vi "AlliGator Load Single Gate Image from .bin File.vi"(6 "Action":T1, 8 "error in (no error)":errorcluster, 10 "File Info":variant, 11 "Gate Index":i32) -> (0 "error out":errorcluster, 1 "Data 2":sgl[][](array[numeric]), 3 "Data 1":sgl[][](array[numeric]))   [LabVIEW 2021, in "AlliGator Files.lvlib"]
doc: "Single gate image loading step for PicoQuant .bin files."
uses:
  AlliGator Files.lvlib
  AlliGator FLI Image Stack Action.ctl
  PicoQuant/BIN/Extended PQ .bin Dataset Information.ctl
  PicoQuant/BIN/BIN File Information.ctl
  PicoQuant/PicoQuant.lvlib
  AlliGator HDF5.lvlib
panel:
  # "see the AlliGator License on the block diagram (Ctrl+E or Window:Show Block Diagram)"
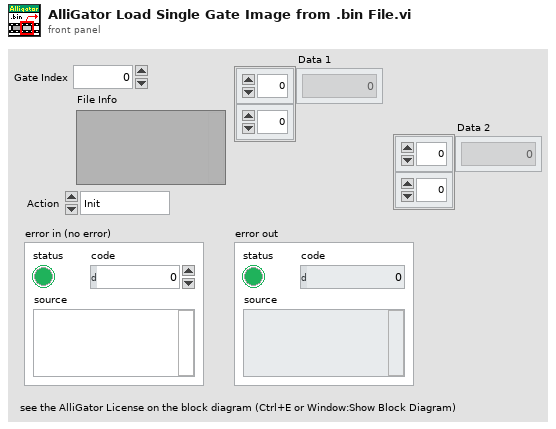
[diagram p1: front panel]
types:
  T1 = typedef "AlliGator HDF5.lvlib/AlliGator FLI Image Stack Action.ctl" = enum16{"Init", "Get Image", "Close"}
  T2 = typedef "PicoQuant.lvlib/Extended PQ .bin Dataset Information.ctl" = cluster{"File Path":path, "offset (in bytes)":i64, "BIN dataset Information":T3}
  T3 = typedef "PicoQuant.lvlib/BIN File Information.ctl" = cluster{"# Pixels X":i32, "# Pixels Y":i32, "Spatial Resolution":dbl[unit], "# TCSPC Bins":i32, "Temporal Resolution":dbl[unit]}
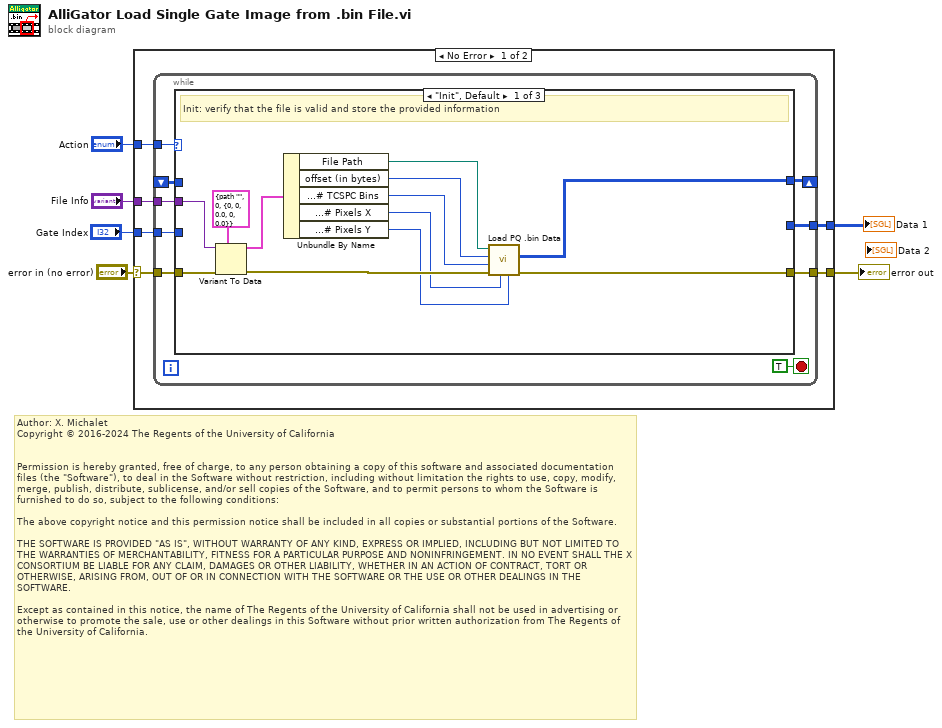
[diagram p0: block diagram]
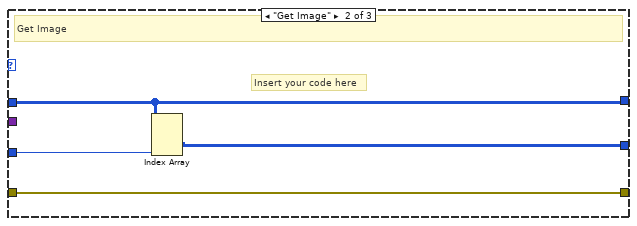
[diagram p2: hidden frame]
diagram:
  # "Author: X. Michalet\nCopyright © 2016-2024 The Regents of the University of California\n \n\nPermission is hereby granted, free of charge, to any person obtaining a copy of this software and associated documentation files (the \"Software\"), to deal in the Software without restriction, including without limitation the rights to use, copy, modify, merge, publish, distribute, sublicense, and/or sell copies of the Software, and to permit persons to whom the Software is furnished to do so, subject to the following conditions:\n\nThe above copyright notice and this permission notice shall be included in all copies or substantial portions of the Software.\n\nTHE SOFTWARE IS PROVIDED \"AS IS\", WITHOUT WARRANTY OF ANY KIND, EXPRESS OR IMPLIED, INCLUDING BUT NOT LIMITED TO THE WARRANTIES OF MERCHANTABILITY, FITNESS FOR A PARTICULAR PURPOSE AND NONINFRINGEMENT. IN NO EVENT SHALL THE X CONSORTIUM BE LIABLE FOR ANY CLAIM, DAMAGES OR OTHER LIABILITY, WHETHER IN AN ACTION OF CONTRACT, TORT OR OTHERWISE, ARISING FROM, OUT OF OR IN CONNECTION WITH THE SOFTWARE OR THE USE OR OTHER DEALINGS IN THE SOFTWARE.\n\nExcept as contained in this notice, the name of The Regents of the University of California shall not be used in advertising or otherwise to promote the sale, use or other dealings in this Software without prior written authorization from The Regents of the University of California."
  n1 = case shown="No Error" "error in (no error)" {
    selector: "error in (no error)" -> [w11 w39]
    tunnel: [w10 w39] -> w5
    tunnel: "Action" -> [w12 _]
    tunnel: "File Info" -> [w9 _]
    tunnel: "Gate Index" -> [w8 _]
    tunnel: [w7 _] -> w1
    frame No Error {
      n2 = while {
        tunnel: w12 -> [w20]
        tunnel: w11 -> [w19]
        tunnel: [w18] -> w10
        tunnel: w9 -> [w17]
        tunnel: w8 -> [w16]
        tunnel: [w15] -> w7
        shift-right: [w14] -> _
        shift-left: _ -> [w13]
        stop <- TRUE stop-if-true
        n3 = case shown="\"Init\", Default" w20 {
          tunnel: w19 -> [w32 w37 w38]
          tunnel: [w30 w37 w38] -> w18
          tunnel: w17 -> [w33 _ _]
          tunnel: w16 -> [_ w35 _]
          tunnel: [_ w34 _] -> w15
          tunnel: [w29 w36 _] -> w14
          tunnel: w13 -> [_ w36 _]
          frame "Init", Default {
            # "Init: verify that the file is valid and store the provided information"
            n4 = Variant To Data(error in=w32, type=T2 {"File Path"=path "", "offset (in bytes)"=0, "BIN dataset Information"={"# Pixels X"=0, "# Pixels Y"=0, "Spatial Resolution"=0.0, "# TCSPC Bins"=0, "Temporal Resolution"=0.0}} ("Extended PQ BIN Dataset Information"), Variant=w33) -> (data=w27:T2, error out=w31:errorcluster)
            n5 = Unbundle By Name(w27) -> ("File Path"=w26:path, "offset (in bytes)"=w25:i64, "BIN dataset Information.# TCSPC Bins"=w24:i32, "BIN dataset Information.# Pixels X"=w23:i32, "BIN dataset Information.# Pixels Y"=w22:i32)
            n6 = call "Load PQ .bin Data.vi"("# Pixels Y"=w22, "# Pixels X"=w23, "error in (no error)"=w31, "# TCSPC Bins"=w24, "offset"=w25, "path in"=w26) -> ("error out"=w30:errorcluster, "Array"=w29:i32[][][])  [unwired: 3 in, 1 out]
          }
          frame "Get Image" {
            # "Insert your code here"
            # "Get Image"
            n7 = Index Array(array=w36, index (dim 2)=w35) -> (element=w34:i32[][])  [unwired: 2 in]
          }
          frame "Close" {
            # "Close File"
          }
        }
      }
    }
    frame Error {
    }
  }
  "Data 1" <- w1
  "error out" <- w5
